vi "Setup subWorker - ModuleC.vi"(8 "error in":errorcluster, 11 "MainUI in":refnum<class "MainUI.lvclass">) -> (0 "error out":errorcluster, 3 "MainUI out":refnum<class "MainUI.lvclass">)   [LabVIEW 2024, in "MainUI.lvclass"]
doc: "This VI sets up the framework parameters of a statically-linked subWorker."
uses:
  MainUI.lvclass
  MainUI.lvclass/MainUI.ctl
  ModuleC/ModuleC.lvclass
  C:/Program Files (x86)/National Instruments/LabVIEW 2024/vi.lib/addons/_Workers/Library/Classes/Worker/Worker.lvclass
  C:/Program Files (x86)/National Instruments/LabVIEW 2024/vi.lib/addons/_Workers/Library/Classes/Workers Object/Workers Object.lvclass
  C:/Users/chrismadlax/Desktop/LVSampleCode/WorkersSchduleDemo/Workers/ModuleC/ModuleC.lvclass
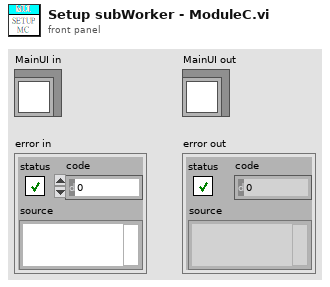
[diagram p1: front panel]
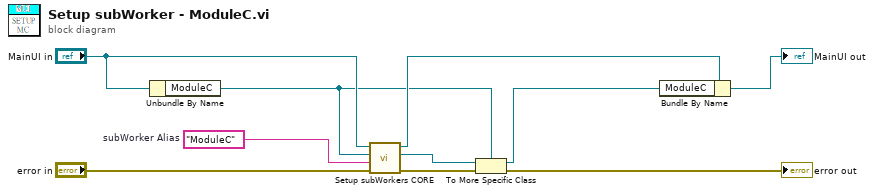
[diagram p0: block diagram]
diagram:
  w6 = "ModuleC"  # subWorker Alias
  n1 = Unbundle By Name("MainUI in") -> ("ModuleC"=w3:refnum<class "ModuleC.lvclass">)
  n2 = call-dynamic "Setup subWorkers CORE.vi"("error in"="error in", "subWorker Alias"=w6, "subWorker"=w3, "Worker"="MainUI in") -> ("error out"=w5:errorcluster, "subWorker out"=w1:refnum<class "Worker.lvclass">, "Worker out"=w8:refnum<class "MainUI.lvclass">)  [unwired: 5 in]
  n3 = To More Specific Class(target class=w3, reference=w1, error in=w5) -> (specific class reference=w2:refnum<class "ModuleC.lvclass">, error out=→"error out":errorcluster)
  n4 = Bundle By Name(cluster=w8, "ModuleC"=w2) -> (→"MainUI out":refnum<class "MainUI.lvclass">)
